vi "Get Data Version.vi"(8 "error in (no error)":errorcluster, 11 "UDP Rx Transfer Configuration in":refnum<class "UDP Transfer Rx Configuration.lvclass">) -> (0 "error out":errorcluster, 2 "data version":T1, 3 "UDP Rx Transfer Configuration out":refnum<class "UDP Transfer Rx Configuration.lvclass">)   [LabVIEW 2023, in "UDP.lvlib" / "UDP Transfer Rx Configuration.lvclass"]
uses:
  UDP Transfer Rx Configuration.lvclass
  Users/Public/Documents/National Instruments/NI VeriStand 2023/Custom Devices/Data Sharing Framework/Linux_x64/DSF Core.lvlibp/Typedefs/DSF Version Info.ctl
  Users/Public/Documents/National Instruments/NI VeriStand 2023/Custom Devices/Data Sharing Framework/Linux_x64/DSF Core.lvlibp
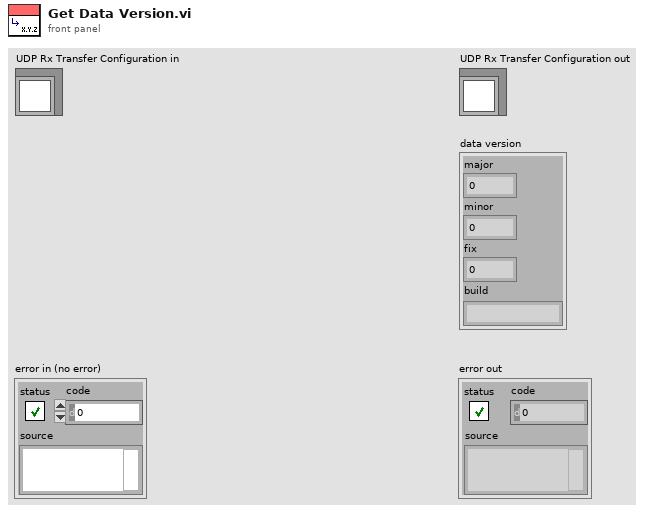
[diagram p1: front panel]
types:
  T1 = typedef "DSF Core.lvlibp/DSF Version Info.ctl" = cluster{"major":u32, "minor":u32, "fix":u32, "build":string}
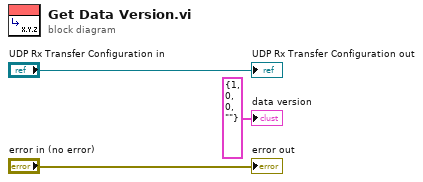
[diagram p0: block diagram]
diagram:
  "error out" <- "error in (no error)"
  "UDP Rx Transfer Configuration out" <- "UDP Rx Transfer Configuration in"
  "data version" <- T1 {"major"=1, "minor"=0, "fix"=0, "build"=""} ("data version")
